vi "Run.vi"(8 "error in (no error)":errorcluster, 9 "s on last turn":dbl, 10 "Maze (0: Empty, -1: Enemy. >0: Teammate":i32[][](array[numeric]), 11 "Spawn in":refnum<class "Spawn.lvclass">) -> (0 "error out":errorcluster, 1 "Direction":T1, 2 "Action":T2, 3 "Spawn out":refnum<class "Spawn.lvclass">, 4 "Replicated":refnum<class "Square.lvclass">)   [LabVIEW 2015, in "Spawn.lvclass"]
uses:
  Spawn.lvclass
  Type Defs/Action Enum.ctl
  Type Defs/Direction Enum.ctl
  Square/Square.lvclass
  Square/Square.lvclass/Square.ctl
  Spawn.lvclass/Spawn.ctl
  Attack/Attack.lvclass
  Attack/Attack.lvclass/Attack.ctl
  Attack/Write Deviation.vi
  Attack/Write Direction.vi
  Attack/Write Frequency.vi
  Square/Read Board Size.vi
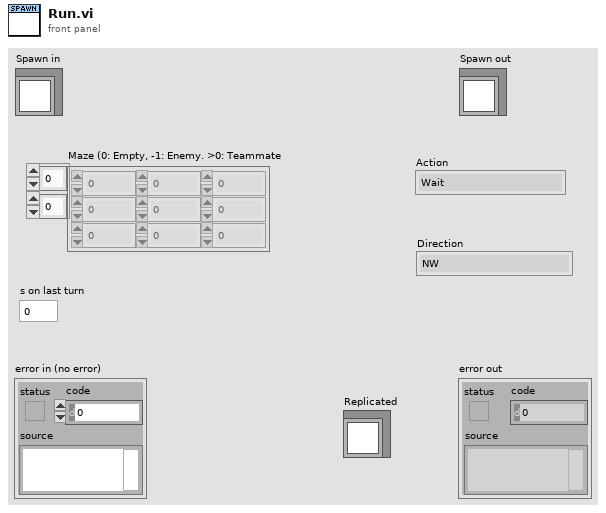
[diagram p1: front panel]
types:
  T1 = typedef "Square.lvclass/Direction Enum.ctl" = enum16{"NW", "N", "NE", "E", "SE", "S", "SW", "W"}
  T2 = typedef "Square.lvclass/Action Enum.ctl" = enum16{"Wait", "Move", "Attack", "Replicate"}
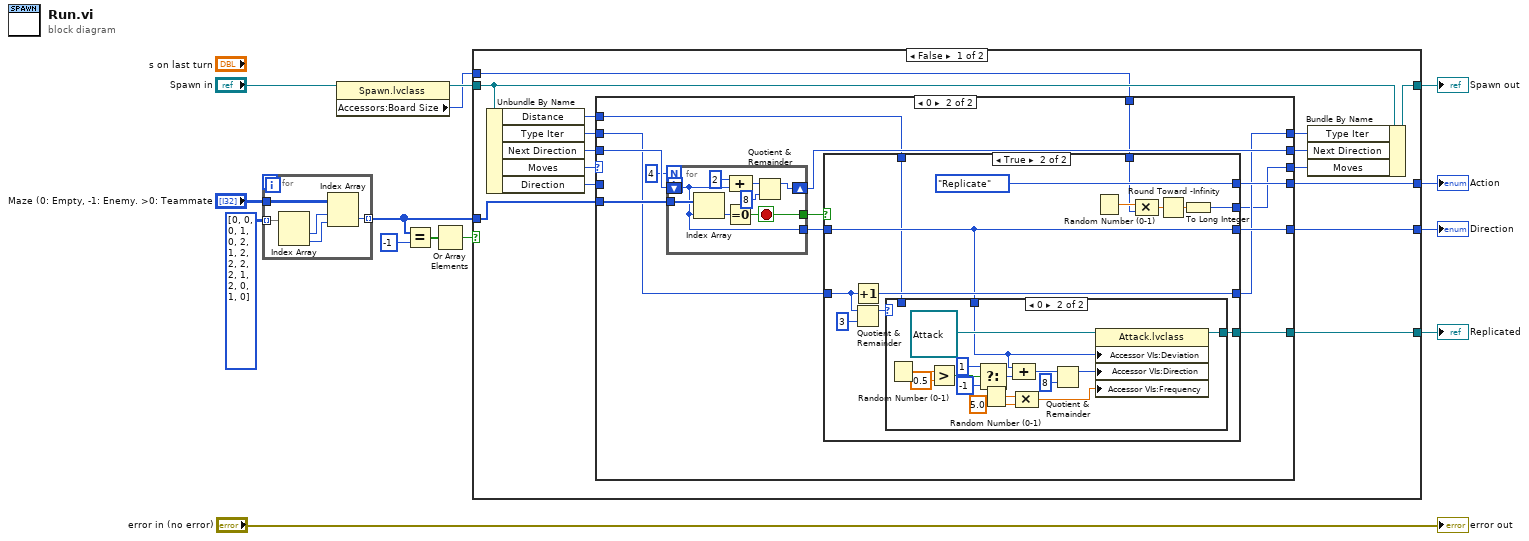
[diagram p0: block diagram]
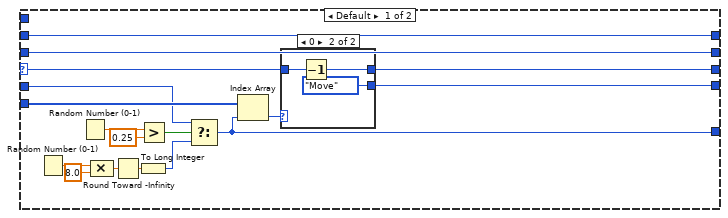
[diagram p2: hidden frame]
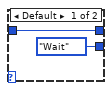
[diagram p3: hidden frame]
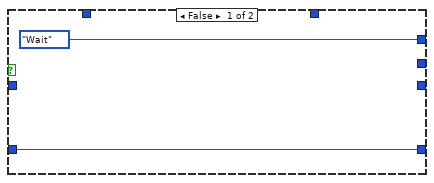
[diagram p4: hidden frame]
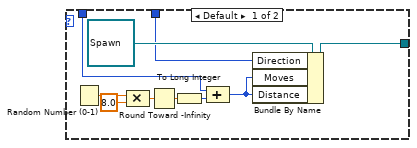
[diagram p5: hidden frame]
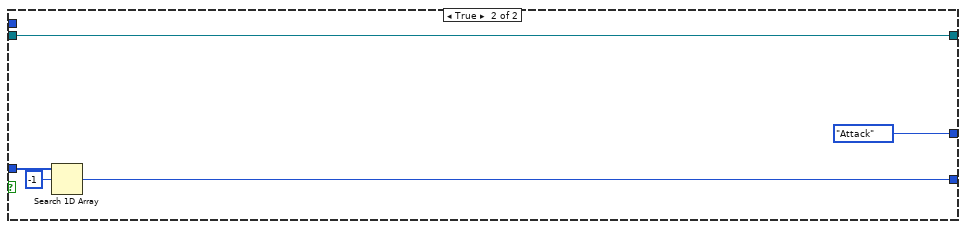
[diagram p6: hidden frame]
diagram:
  n1 = for {
    tunnel: "Maze (0: Empty, -1: Enemy. >0: Teammate" -> [w19]
    tunnel: i32[][] [[0, 0], [0, 1], [0, 2], [1, 2], [2, 2], [2, 1], [2, 0], [1, 0]] -> [w18] mode=indexing
    tunnel: [w15] -> w6 mode=indexing
    n2 = Index Array(array=w18) -> (element #1=w17:i32, element #2=w16:i32)  [unwired: 2 in]
    n3 = Index Array(array=w19, index (row)=w17, index (col)=w16) -> (element=w15:i32)
  }
  n4 = property class="Spawn.lvclass"(reference="Spawn in") -> (reference out=w2:refnum<class "Spawn.lvclass">, "Accessors:Board Size"=w1:i32)  [unwired: 1 in, 1 out]
  n5 = Equal?(x=w6, y=-1) -> (x = y?=w5:bool[])
  n6 = Or Array Elements(Boolean array=w5) -> (logical OR=w4:bool)
  n7 = case shown="False" w4 {
    tunnel: [w34 Action_Enum."Attack" ("Action")] -> w13
    tunnel: w2 -> [w32 w123]
    tunnel: [w31 w123] -> w12
    tunnel: [w29 w119] -> w11
    tunnel: [w27 _] -> w10
    tunnel: w6 -> [w24 w121]
    tunnel: w1 -> [w20 _]
    frame False {
      n8 = Unbundle By Name(w32) -> ("Distance"=w21:i32, "Type Iter"=w23:i32, "Next Direction"=w26:T1, "Moves"=w33:i32, "Direction"=w28:T1)
      n9 = case shown="0" w33 {
        selector: w33 -> [w51 _]
        tunnel: [w49 w70] -> w34
        tunnel: [w50 w58] -> w30
        tunnel: w28 -> [w36 _]
        tunnel: [w35 w69] -> w29
        tunnel: [_ w68] -> w27
        tunnel: w26 -> [w47 w67]
        tunnel: [w47 w66] -> w25
        tunnel: w24 -> [w46 w65]
        tunnel: w23 -> [w45 w64]
        tunnel: [w45 w63] -> w22
        tunnel: w21 -> [_ w59]
        tunnel: w20 -> [_ w57]
        frame Default {
          n10 = Random Number (0-1)() -> (number: 0 to 1=w42:dbl)
          n11 = Random Number (0-1)() -> (number: 0 to 1=w44:dbl)
          n12 = Compound Arithmetic op=MULTIPLY(w42, 8.0 ("value")) -> (w40:dbl)
          n13 = Round Toward -Infinity(1:w40) -> (0:w38:dbl)
          n14 = To Long Integer(number=w38) -> (32bit integer=w37:i32)
          n15 = Greater?(x=w44, y=0.25) -> (0:w39:bool)
          n16 = Select(t=w36, s=w39, f=w37) -> (s? t:f=w35:i32)
          n17 = Index Array(array=w46, index=w35) -> (element=w48:i32)
          n18 = case shown="0" w48 {
            tunnel: w51 -> [w53 w56]
            tunnel: [w53 w55] -> w50
            tunnel: [Action_Enum."Wait" ("Action") Action_Enum."Move" ("Action")] -> w49
            frame Default {
            }
            frame 0 {
              n19 = Decrement(x=w56) -> (x-1=w55:i32)
            }
          }
        }
        frame 0 {
          n20 = for {
            N: 4 -> [_]
            tunnel: w65 -> [w118]
            tunnel: [w116] -> w61
            shift-right: [w113] -> w66
            shift-left: w67 -> [w111]
            tunnel: [w111] -> w60
            stop <- w116 stop-if-true
            n21 = Index Array(array=w118, index=w111) -> (element=w117:i32)
            n22 = Equal To 0?(x=w117) -> (x = 0?=w116:bool)
            n23 = Compound Arithmetic op=ADD(2, w111) -> (w114:i32)
            n24 = Quotient & Remainder(x=w114, y=8) -> (x-y*floor(x/y)=w113:i32)  [unwired: 1 out]
          }
          n25 = case shown="True" w61 {
            tunnel: [Action_Enum."Wait" ("Action") Action_Enum."Replicate" ("Action")] -> w70
            tunnel: [_ w79] -> w69
            tunnel: w60 -> [_ w79]
            tunnel: w64 -> [w71 w83]
            tunnel: [w71 w82] -> w63
            tunnel: [_ w80] -> w68
            tunnel: w59 -> [_ w78]
            tunnel: [_ w74] -> w58
            tunnel: w57 -> [_ w73]
            frame False {
            }
            frame True {
              n26 = Increment(x=w83) -> (x+1=w82:i32)
              n27 = Quotient & Remainder(x=w83, y=3) -> (x-y*floor(x/y)=w81:i32)  [unwired: 1 out]
              n28 = case shown="0" w81 {
                tunnel: [w94 w109] -> w80
                tunnel: w79 -> [w93 w105]
                tunnel: w78 -> [w86 _]
                frame Default {
                  n29 = Random Number (0-1)() -> (number: 0 to 1=w92:dbl)
                  n30 = Compound Arithmetic op=MULTIPLY(w92, 8.0 ("value")) -> (w90:dbl)
                  n31 = Round Toward -Infinity(1:w90) -> (0:w89:dbl)
                  n32 = To Long Integer(number=w89) -> (32bit integer=w88:i32)
                  n33 = Compound Arithmetic op=ADD(w86, w88) -> (w87:i32)
                  n34 = Bundle By Name(cluster=refnum<class "Spawn.lvclass"> refnum ("Spawn.lvclass"), "Direction"=w93, "Moves"=w87, "Distance"=w87) -> (w94:refnum<class "Spawn.lvclass">)
                }
                frame 0 {
                  n35 = Random Number (0-1)() -> (number: 0 to 1=w108:dbl)
                  n36 = Greater?(x=w108, y=0.5) -> (0:w106:bool)
                  n37 = Select(t=1, s=w106, f=-1) -> (s? t:f=w104:i32)
                  n38 = Random Number (0-1)() -> (number: 0 to 1=w98:dbl)
                  n39 = Compound Arithmetic op=ADD(w105, w104) -> (w101:i32)
                  n40 = Compound Arithmetic op=MULTIPLY(w98, 5.0 ("value")) -> (w96:dbl)
                  n41 = Quotient & Remainder(x=w101, y=8) -> (x-y*floor(x/y)=w100:i32)  [unwired: 1 out]
                  n42 = property class="Attack.lvclass"(reference=refnum<class "Attack.lvclass"> refnum ("Attack.lvclass"), "Accessor VIs:Deviation"=w105, "Accessor VIs:Direction"=w100, "Accessor VIs:Frequency"=w96) -> (reference out=w109:refnum<class "Attack.lvclass">)  [unwired: 1 in, 1 out]
                }
              }
              n43 = Random Number (0-1)() -> (number: 0 to 1=w75:dbl)
              n44 = Compound Arithmetic op=MULTIPLY(w75, w73) -> (w76:dbl)
              n45 = Round Toward -Infinity(1:w76) -> (0:w77:dbl)
              n46 = To Long Integer(number=w77) -> (32bit integer=w74:i32)
            }
          }
        }
      }
      n47 = Bundle By Name(cluster=w32, "Type Iter"=w22, "Next Direction"=w25, "Moves"=w30) -> (w31:refnum<class "Spawn.lvclass">)
    }
    frame True {
      n48 = Search 1D Array(1D array=w121, element=-1) -> (index of element=w119:i32)  [unwired: 1 in]
    }
  }
  "Spawn out" <- w12
  "Action" <- w13
  "Direction" <- w11
  "Replicated" <- w10
  "error out" <- "error in (no error)"
